vi "Measuring_Instrument.vi"(0 "Write String":string, 5 "Read String":string) -> (4 "Readed Data":string)   [LabVIEW 2020]
doc: "This is the SubVI which is used to get in data from the input instrument and introducing an error in the input and saving it in the file"
uses:
  <vilib>/Utility/config.llb/Read Key (String).vi
  <vilib>/Utility/config.llb/Write Key (String).vi
  <vilib>/Utility/config.llb/NI_LVConfig.lvlib
panel:
  out "Read error":errorcluster
  out "Write error":errorcluster
  # "OUTPUT"
  # "INPUT"
  # "This VI gets in values introduces error and returns it if specified input is given"
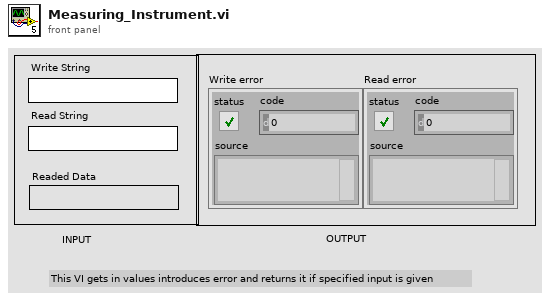
[diagram p1: front panel]
types:
  T1 = typedef "NI_LVConfig.lvlib/Config Data RefNum.ctl" = refnum<k1>
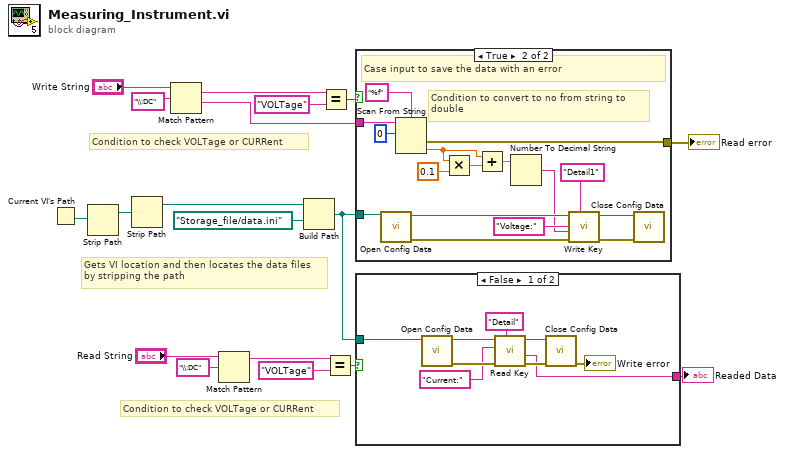
[diagram p0: block diagram]
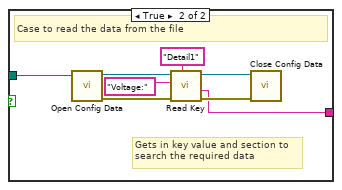
[diagram p2: hidden frame]
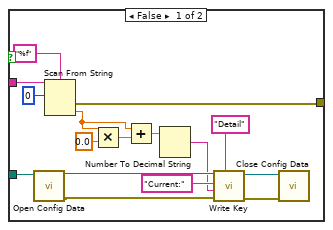
[diagram p3: hidden frame]
diagram:
  # "Condition to check VOLTage or CURRent"
  # "Condition to check VOLTage or CURRent"
  # "Gets VI location and then locates the data files\nby stripping the path"
  n1 = Current VI's Path() -> (path=w8:path)
  n2 = Strip Path(path=w8) -> (stripped path=w7:path)  [unwired: 1 out]
  n3 = Strip Path(path=w7) -> (stripped path=w6:path)  [unwired: 1 out]
  n4 = Match Pattern(string="Write String", regular expression="\\:DC") -> (before substring=w17:string, after substring=w2:string)  [unwired: 1 in, 2 out]
  n5 = Match Pattern(string="Read String", regular expression="\\:DC") -> (before substring=w12:string)  [unwired: 1 in, 3 out]
  n6 = Build Path(base path=w6, name or relative path=path "Storage_file/data.ini") -> (appended path=w4:path)
  n7 = Equal?(x=w17, y="VOLTage") -> (x = y?=w15:bool)
  n8 = Equal?(x=w12, y="VOLTage") -> (x = y?=w9:bool)
  n9 = case shown="True" w15 {
    tunnel: w4 -> [w32 w48]
    tunnel: w2 -> [w31 w43]
    tunnel: [w19 w36] -> w1
    frame False {
      n10 = call <vilib>:"Open Config Data.vi"("configuration file path"=w32) -> ("error out"=w22:errorcluster, "refnum"=w23:T1)  [unwired: 8 in, 1 out]
      n11 = Scan From String(format string="%f", input string=w31, initial scan location=u32 0) -> (error out=w19:errorcluster, output 1=w26:dbl)  [unwired: 2 in, 2 out]
      n12 = Multiply(x=w26, y=0.0) -> (x*y=w27:dbl)
      n13 = Add(x=w26, y=w27) -> (x+y=w25:dbl)
      n14 = Number To Decimal String(number=w25) -> (decimal integer string=w21:string)  [unwired: 1 in]
      n15 = call-poly <vilib>:"Write Key.vi"("section"="Detail", "error in (no error)"=w22, "value"=w21, "key"="Current:" ("string"), "refnum"=w23) -> ("error out"=w33:errorcluster, "refnum out"=w34:T1)  [unwired: 4 in, 1 out]
      n16 = call <vilib>:"Close Config Data.vi"("error in (no error)"=w33, "refnum"=w34) -> ()  [unwired: 8 in, 2 out]
    }
    frame True, Default {
      # "Condition to convert to no from string to\ndouble"
      # "Case input to save the data with an error"
      n17 = call <vilib>:"Open Config Data.vi"("configuration file path"=w48) -> ("error out"=w40:errorcluster, "refnum"=w41:T1)  [unwired: 8 in, 1 out]
      n18 = Scan From String(format string="%f", input string=w43, initial scan location=u32 0) -> (error out=w36:errorcluster, output 1=w35:dbl)  [unwired: 2 in, 2 out]
      n19 = Multiply(x=w35, y=0.1) -> (x*y=w46:dbl)
      n20 = Add(x=w35, y=w46) -> (x+y=w45:dbl)
      n21 = Number To Decimal String(number=w45) -> (decimal integer string=w38:string)  [unwired: 1 in]
      n22 = call-poly <vilib>:"Write Key.vi"("section"="Detail1", "error in (no error)"=w40, "value"=w38, "key"="Voltage:" ("string"), "refnum"=w41) -> ("error out"=w49:errorcluster, "refnum out"=w50:T1)  [unwired: 4 in, 1 out]
      n23 = call <vilib>:"Close Config Data.vi"("error in (no error)"=w49, "refnum"=w50) -> ()  [unwired: 8 in, 2 out]
    }
  }
  "Read error" <- w1
  n24 = case shown="False" w9 {
    tunnel: w4 -> [w58 w65]
    tunnel: [w51 w61] -> w3
    frame False {
      n25 = call <vilib>:"Open Config Data.vi"("configuration file path"=w58) -> ("error out"=w59:errorcluster, "refnum"=w54:T1)  [unwired: 8 in, 1 out]
      n26 = call-poly <vilib>:"Read Key.vi"("section"="Detail", "error in (no error)"=w59, "key"="Current:", "refnum"=w54) -> ("error out"=w56:errorcluster, "value"=w51:string, "refnum out"=w55:T1)  [unwired: 4 in, 1 out]
      n27 = call <vilib>:"Close Config Data.vi"("error in (no error)"=w56, "refnum"=w55) -> ("error out"=→"Write error":errorcluster)  [unwired: 8 in, 1 out]
    }
    frame True {
      # "Gets in key value and section to\nsearch the required data"
      # "Case to read the data from the file"
      n28 = call <vilib>:"Open Config Data.vi"("configuration file path"=w65) -> ("error out"=w66:errorcluster, "refnum"=w67:T1)  [unwired: 8 in, 1 out]
      n29 = call-poly <vilib>:"Read Key.vi"("section"="Detail1", "error in (no error)"=w66, "key"="Voltage:", "refnum"=w67) -> ("error out"=w63:errorcluster, "value"=w61:string, "refnum out"=w64:T1)  [unwired: 4 in, 1 out]
      n30 = call <vilib>:"Close Config Data.vi"("error in (no error)"=w63, "refnum"=w64) -> ()  [unwired: 8 in, 2 out]
    }
  }
  "Readed Data" <- w3
